vi "Sprawdz sasiedztwo.vi"(8 "error in (no error)":errorcluster, 10 "Position":T1, 11 "Array of boids":refnum<class "Boid.lvclass">[](array[class])) -> (2 "Sasiedzi":i32[](array[numeric]))   [LabVIEW 2014, in "Swiat.lvclass"]
uses:
  Swiat.lvclass
  Typedefs/Position.ctl
  Boid/Boid.lvclass
  Boid/Boid.lvclass/Boid.ctl
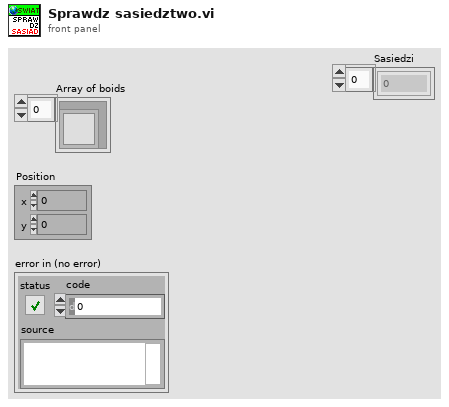
[diagram p1: front panel]
types:
  T1 = typedef "Position.ctl" = cluster{"x":i16, "y":i16}
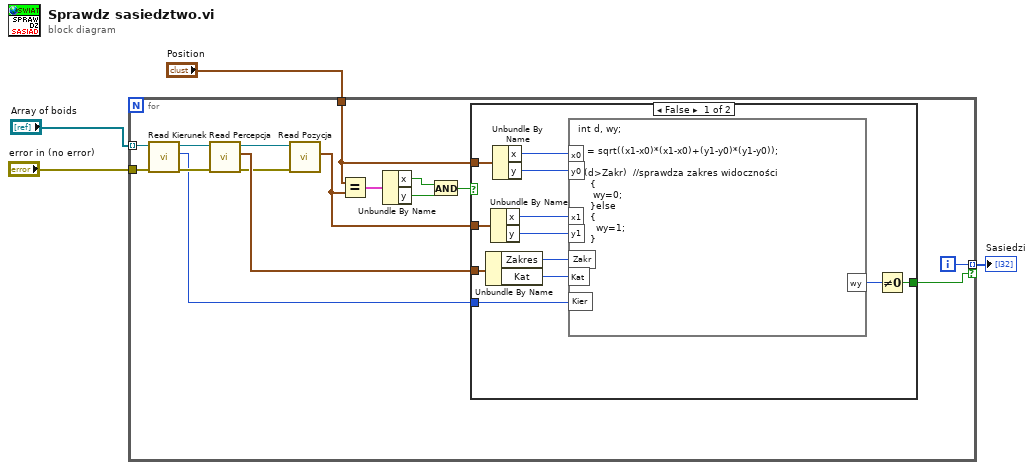
[diagram p0: block diagram]
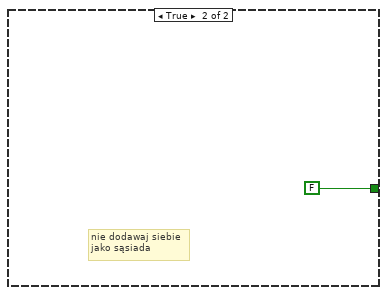
[diagram p2: hidden frame]
diagram:
  n1 = for {
    tunnel: "Array of boids" -> [w8] mode=indexing
    tunnel: "error in (no error)" -> [w9]
    tunnel: "Position" -> [w16]
    tunnel: [w14] -> w1 mode=indexing if=w13
    i -> [w14]
    n2 = call "Read Kierunek.vi"("error in (no error)"=w9, "Boid in"=w8) -> ("error out"=w7:errorcluster, "Kierunek"=w5:i16, "Boid out"=w6:refnum<class "Boid.lvclass">)  [unwired: 7 in]
    n3 = call "Read Percepcja.vi"("error in (no error)"=w7, "Boid in"=w6) -> ("error out"=w11:errorcluster, "Percepcja"=w12:cluster{"Zakres":i16, "Kat":i16}, "Boid out"=w10:refnum<class "Boid.lvclass">)  [unwired: 7 in]
    n4 = call "Read Pozycja.vi"("error in (no error)"=w11, "Boid in"=w10) -> ("Position"=w15:T1)  [unwired: 7 in, 2 out]
    n5 = Equal?(x=w16, y=w15) -> (x = y?=w20:cluster{"x":bool, "y":bool})
    n6 = Unbundle By Name(w20) -> ("x"=w18:bool, "y"=w19:bool)
    n7 = And(x=w18, y=w19) -> (x .and. y?=w17:bool)
    n8 = case shown="False" w17 {
      tunnel: w16 -> [w31 _]
      tunnel: w15 -> [w32 _]
      tunnel: [w24 FALSE] -> w13
      tunnel: w12 -> [w26 _]
      tunnel: w5 -> [w21 _]
      frame False {
        n9 = Unbundle By Name(w26) -> ("Zakres"=w25:i16, "Kat"=w22:i16)
        n10 = Unbundle By Name(w32) -> ("x"=w28:i16, "y"=w27:i16)
        n11 = Unbundle By Name(w31) -> ("x"=w30:i16, "y"=w29:i16)
        n12 = formula code="int d, wy;\n\nd = sqrt((x1-x0)*(x1-x0)+(y1-y0)*(y1-y0));\n\nif(d>Zakr)  //sprawdza zakres widoczności\n    {\n     wy=0;\n    }else\n    {\n      wy=1;\n    }"("x0"=w30, "y0"=w29, "x1"=w28, "y1"=w27, "Zakr"=w25, "Kat"=w22, "Kier"=w21) -> ("wy"=w23:i32)
        n13 = Not Equal To 0?(x=w23) -> (x != 0?=w24:bool)
      }
      frame True {
        # "nie dodawaj siebie\njako sąsiada"
      }
    }
  }
  "Sasiedzi" <- w1
